vi "Initialize Hardware.vi"(7 "RT config file":path, 8 "error in":errorcluster, 11 "device parameters":T5) -> (0 "error out":errorcluster, 3 "RT handles":T4, 5 "device information":T1)   [LabVIEW 2020, in "Ballard ARINC 429 Engine.lvlib" / "Custom Device.lvlib"]
uses:
  Custom Device.lvlib
  <instrlib>/BTICardLib/BTICardLV.lvlib
  <instrlib>/BTICardLib/Private/IO/Action-Status/Write External LED.vi
  <instrlib>/BTI429Lib/BTI429LV.lvlib
  Shared/Direction Capability.ctl
  Hardware Direction and Channels.ctl
  Device Information.ctl
  Hardware Handles.ctl
  <instrlib>/BTICardLib/Private/Initialize By Slot Number and Core Number.vi
  <instrlib>/BTICardLib/Private/Initialize By Card Number and Core Number.vi
  <instrlib>/BTICardLib/Private/Configure All From XML.vi
  <instrlib>/BTI429Lib/Private/Core/Action-Status/Start All Channels.vi
  Shared/Initialization Method.ctl
  Shared/Device Parameters.ctl
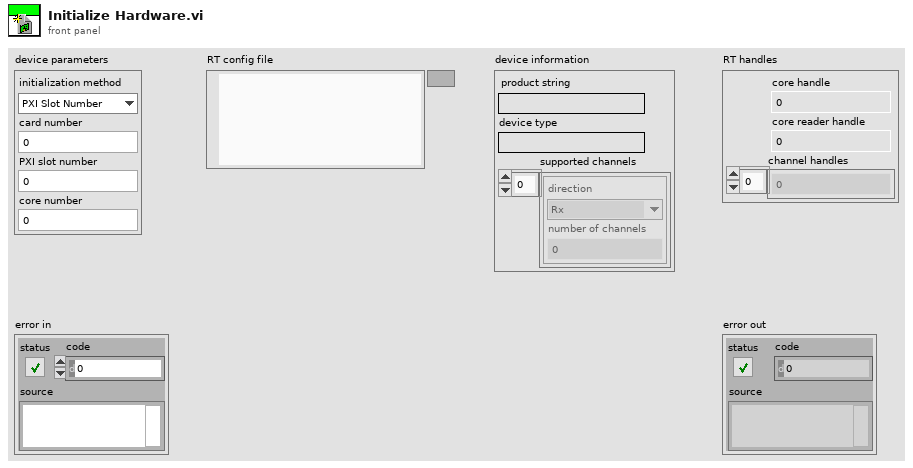
[diagram p1: front panel]
types:
  T1 = typedef "Ballard ARINC 429 Engine.lvlib/Custom Device.lvlib/Device Information.ctl" = cluster{"product string":string, "device type":string, "supported channels":T2[]}
  T2 = typedef "Ballard ARINC 429 Engine.lvlib/Custom Device.lvlib/Hardware Direction and Channels.ctl" = cluster{"direction":T3, "number of channels":u16}
  T3 = typedef "Direction Capability.ctl" = enum16{"Rx", "Tx", "Rx/Tx"}
  T4 = typedef "Ballard ARINC 429 Engine.lvlib/Custom Device.lvlib/Hardware Handles.ctl" = cluster{"core handle":u64, "core reader handle":u64, "channel handles":u64[]}
  T5 = typedef "Device Parameters.ctl" = cluster{"initialization method":T6, "card number":i32, "PXI slot number":i32, "core number":i32}
  T6 = typedef "Initialization Method.ctl" = enum16{"PXI Slot Number", "Card Number"}
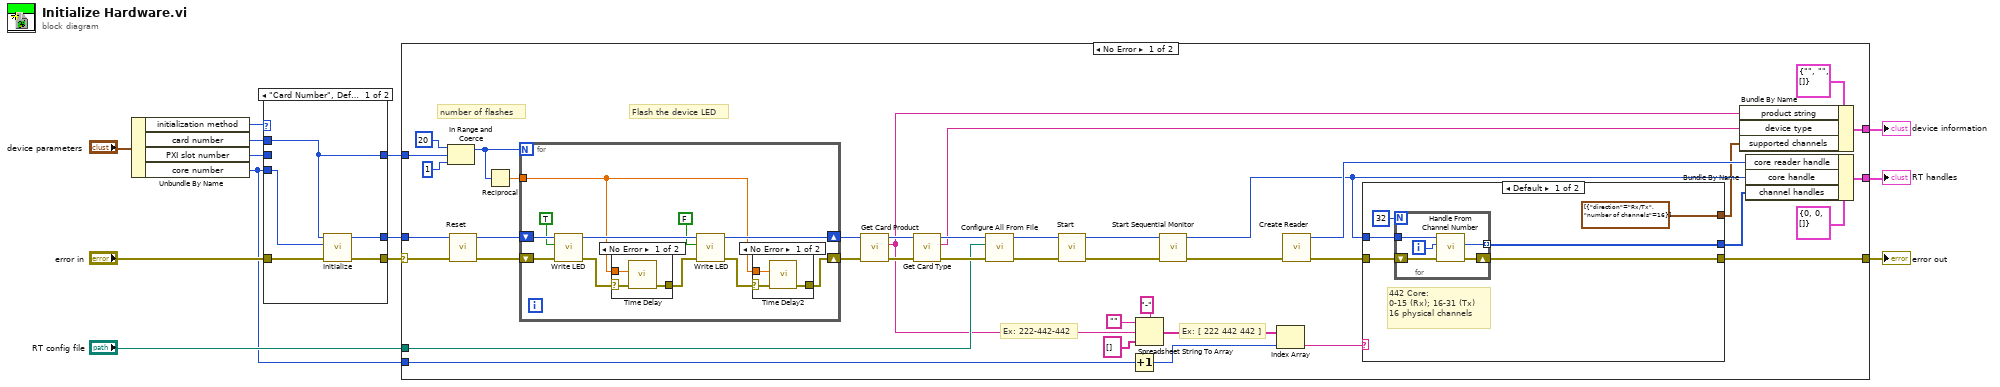
[diagram p0: block diagram]
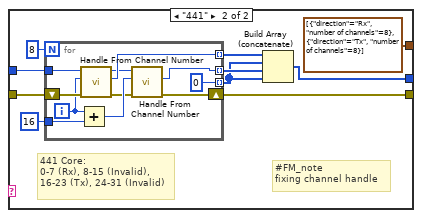
[diagram p2: hidden frame]
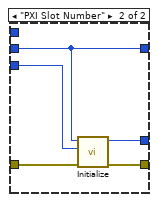
[diagram p6: hidden frame]
diagram:
  n1 = Unbundle By Name("device parameters") -> ("initialization method"=w13:T6, "card number"=w12:i32, "PXI slot number"=w11:i32, "core number"=w1:i32)
  n2 = case shown="\"Card Number\", Default" w13 {
    tunnel: [w18 w23] -> w7
    tunnel: [w17 w22] -> w9
    tunnel: w12 -> [w14 _]
    tunnel: "error in" -> [w16 w21]
    tunnel: w11 -> [_ w19]
    tunnel: w1 -> [w15 w20]
    tunnel: [w14 w19] -> w6
    frame "Card Number", Default {
      n3 = call-poly <instrlib>:"Initialize.vi"("error in (no error)"=w16, "core number"=w15, "card number"=w14) -> ("error out"=w17:errorcluster, "core handle out"=w18:u64)  [unwired: 7 in]
    }
    frame "PXI Slot Number" {
      n4 = call-poly <instrlib>:"Initialize.vi"("error in (no error)"=w21, "core number"=w20, "slot number"=w19) -> ("error out"=w22:errorcluster, "core handle out"=w23:u64)  [unwired: 7 in]
    }
  }
  n5 = case shown="No Error" w9 {
    selector: w9 -> [w63 w115]
    tunnel: w7 -> [w62 _]
    tunnel: w6 -> [w59 _]
    tunnel: [w40 _] -> w5
    tunnel: [w38 _] -> w4
    tunnel: [w37 w115] -> w3
    tunnel: "RT config file" -> [w34 _]
    tunnel: w1 -> [w26 _]
    frame No Error {
      # "Ex: [ 222 442 442 ]"
      # "Ex: 222-442-442"
      # "number of flashes"
      # "Flash the device LED"
      n6 = In Range and Coerce(upper limit=20 ("x"), x=w59, lower limit=1) -> (coerced(x)=w55:i32)  [unwired: 1 out]
      n7 = call <instrlib>:"Reset.vi"("error in (no error)"=w63, "core handle in"=w62) -> ("error out"=w61:errorcluster, "core handle out"=w60:u64)  [unwired: 8 in]
      n8 = Reciprocal(x=w55) -> (1/x=w56:dbl)
      n9 = for {
        N: w55 -> [_]
        shift-right: [w105] -> w52
        shift-left: w60 -> [w104]
        shift-right: [w99] -> w51
        shift-left: w61 -> [w103]
        tunnel: w56 -> [w96]
        n10 = call-poly <instrlib>:"Write LED.vi"("error in (no error)"=w103, "LED state"=TRUE, "core handle in"=w104) -> ("error out"=w98:errorcluster, "core handle out"=w106:u64)  [unwired: 7 in]
        n11 = case shown="No Error" w98 {
          selector: w98 -> [w109 w110]
          tunnel: [w108 w110] -> w97
          tunnel: w96 -> [w107 _]
          frame No Error {
            n12 = call "Time Delay"("error in (no error)"=w109, "Delay Time (s)"=w107) -> ("error out"=w108:errorcluster)  [unwired: 9 in]
          }
          frame Error {
          }
        }
        n13 = call-poly <instrlib>:"Write LED.vi"("error in (no error)"=w97, "LED state"=FALSE, "core handle in"=w106) -> ("error out"=w100:errorcluster, "core handle out"=w105:u64)  [unwired: 7 in]
        n14 = case shown="No Error" w100 {
          selector: w100 -> [w113 w114]
          tunnel: [w112 w114] -> w99
          tunnel: w96 -> [w111 _]
          frame No Error {
            n15 = call "Time Delay2"("error in (no error)"=w113, "Delay Time (s)"=w111) -> ("error out"=w112:errorcluster)  [unwired: 9 in]
          }
          frame Error {
          }
        }
      }
      n16 = call <instrlib>:"Get Card Product.vi"("error in (no error)"=w51, "core handle in"=w52) -> ("error out"=w53:errorcluster, "product string out"=w28:string, "core handle out"=w54:u64)  [unwired: 7 in]
      n17 = call <instrlib>:"Get Card Type.vi"("error in (no error)"=w53, "core handle in"=w54) -> ("error out"=w43:errorcluster, "type string out"=w42:string, "core handle out"=w44:u64)  [unwired: 7 in]
      n18 = call-poly <instrlib>:"Configure All From File.vi"("error in (no error)"=w43, "configuration file path"=w34, "core handle in"=w44) -> ("error out"=w46:errorcluster, "core handle out"=w47:u64)  [unwired: 7 in]
      n19 = call-poly <instrlib>:"Start.vi"("error in (no error)"=w46, "core handle in"=w47) -> ("error out"=w49:errorcluster, "core handle out"=w48:u64)  [unwired: 8 in]
      n20 = Increment(x=w26) -> (x+1=w29:i32)
      n21 = Spreadsheet String To Array(delimiter (Tab)="-", format string="", spreadsheet string=w28, array type (2D Dbl)=string[] []) -> (array=w30:string[])
      n22 = call <instrlib>:"Start Sequential Monitor.vi"("error in (no error)"=w49, "core handle in"=w48) -> ("error out"=w50:errorcluster, "core handle out"=w33:u64)  [unwired: 8 in]
      n23 = Index Array(array=w30, index=w29) -> (element=w25:string)
      n24 = call <instrlib>:"Create Reader.vi"("error in (no error)"=w50) -> ("error out"=w45:errorcluster, "core reader handle out"=w35:u64)  [unwired: 9 in]
      n25 = case shown="Default" w25 {
        tunnel: w45 -> [w68 w83]
        tunnel: [w67 w82] -> w37
        tunnel: [w66 w76] -> w36
        tunnel: w33 -> [w65 w81]
        tunnel: [T2[] [{"direction"=enum."Rx/Tx", "number of channels"=16}] ("supported channels") T2[] [{"direction"=enum."Rx", "number of channels"=8}, {"direction"=enum."Tx", "number of channels"=8}] ("supported channels")] -> w24
        frame Default {
          # "442 Core:\n0-15 (Rx); 16-31 (Tx)\n16 physical channels"
          n26 = for {
            N: 32 -> [_]
            shift-right: [w71] -> w67
            shift-left: w68 -> [w74]
            tunnel: [w72] -> w66 mode=indexing
            tunnel: w65 -> [w70]
            i -> [w73]
            n27 = call <instrlib>:"Handle From Channel Number.vi"("error in (no error)"=w74, "channel number"=w73, "core handle in"=w70) -> ("error out"=w71:errorcluster, "channel handle out"=w72:u64)  [unwired: 6 in, 1 out]
          }
        }
        frame "441" {
          # "#FM_note\nfixing channel handle"
          # "441 Core:\n0-7 (Rx), 8-15 (Invalid),\n16-23 (Tx), 24-31 (Invalid)"
          n28 = for {
            N: 8 -> [_]
            shift-right: [w86] -> w82
            shift-left: w83 -> [w95]
            tunnel: [w94] -> w80 mode=indexing
            tunnel: w81 -> [w93]
            tunnel: [w85] -> w79 mode=indexing
            tunnel: 16 ("y") -> [w89]
            tunnel: [u64 0 ("channel handle out")] -> w77 mode=indexing
            i -> [w91]
            n29 = Add(x=w91, y=w89) -> (x+y=w90:i32)
            n30 = call <instrlib>:"Handle From Channel Number.vi"("error in (no error)"=w95, "channel number"=w91, "core handle in"=w93) -> ("error out"=w87:errorcluster, "channel handle out"=w94:u64, "core handle out"=w92:u64)  [unwired: 6 in]
            n31 = call <instrlib>:"Handle From Channel Number.vi"("error in (no error)"=w87, "channel number"=w90, "core handle in"=w92) -> ("error out"=w86:errorcluster, "channel handle out"=w85:u64)  [unwired: 6 in, 1 out]
          }
          n32 = Build Array (concatenate)(w80, w77, w79, w77) -> (w76:u64[])
        }
      }
      n33 = Bundle By Name(cluster=T1 {"product string"="", "device type"="", "supported channels"=[]} ("hardware information"), "product string"=w28, "device type"=w42, "supported channels"=w24) -> (w40:T1)
      n34 = Bundle By Name(cluster=T4 {"core handle"=0, "core reader handle"=0, "channel handles"=[]} ("hardware handles"), "core reader handle"=w35, "core handle"=w33, "channel handles"=w36) -> (w38:T4)
    }
    frame Error {
    }
  }
  "RT handles" <- w4
  "error out" <- w3
  "device information" <- w5
